vi "Stop.vi"   [LabVIEW 2011]
uses:
  _GlobalVariables&Libraries/ATV Program Global Variables.vi
types:
  T1 = cluster{"Drive Value Output String":string, "Steer Value Output String":string, "Error Out":errorcluster, "Initial Encoder Counts":string, "Disable Galil Terminal":bool, "Command Input":string}
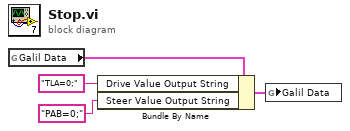
[diagram p0: block diagram]
diagram:
  n1 = global read "ATV Program Global Variables.vi" "Galil Data"() -> (w2:T1)
  n2 = Bundle By Name(cluster=w2, "Drive Value Output String"="TLA=0;", "Steer Value Output String"="PAB=0;") -> (w1:T1)
  n3 = global write "ATV Program Global Variables.vi" "Galil Data"(w1) -> ()
